vi "Replace Nested Parenthesis Pairs.vi"(6 "Existing Variables":string[](array[string]), 8 "Error In":errorcluster, 9 "Array of Parenthesis Pairs":cluster{"Start Index":i32, "Stop Index":i32}[](array[cluster]), 10 "New Variables":string[](array[string]), 11 "Formula String":string) -> (0 "Error Out":errorcluster, 1 "Array of Binary Formulas":T1[](array[typedef]), 2 "Replaced Strings":string[](array[string]), 3 "Formula String (simplified)":string)   [LabVIEW 2021, in "Formula.lvlib"]
uses:
  Binary Formula.ctl
  Binary Formula Step.ctl
  Binary Operator.ctl
  Formula.lvlib
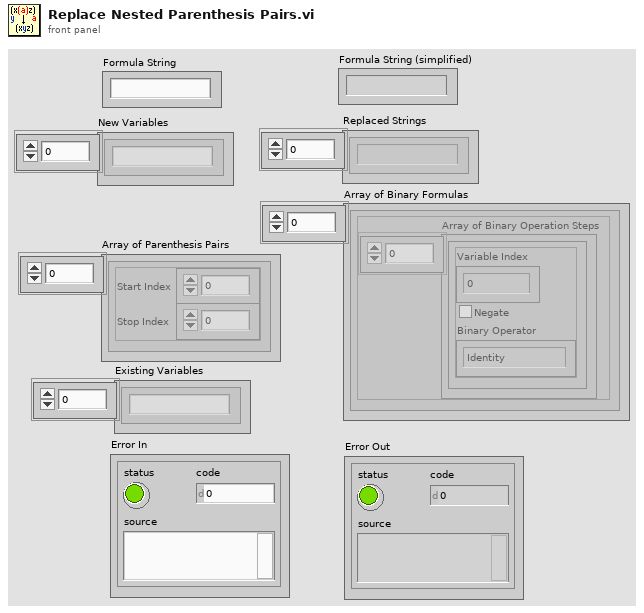
[diagram p1: front panel]
types:
  T1 = typedef "Formula.lvlib/Binary Formula.ctl" = cluster{"Array of Binary Operation Steps":T2[]}
  T2 = typedef "Formula.lvlib/Binary Formula Step.ctl" = cluster{"Variable Index":i32, "Negate":bool, "Binary Operator":T3}
  T3 = typedef "Formula.lvlib/Binary Operator.ctl" = enum16{"Identity", "AND", "OR"}
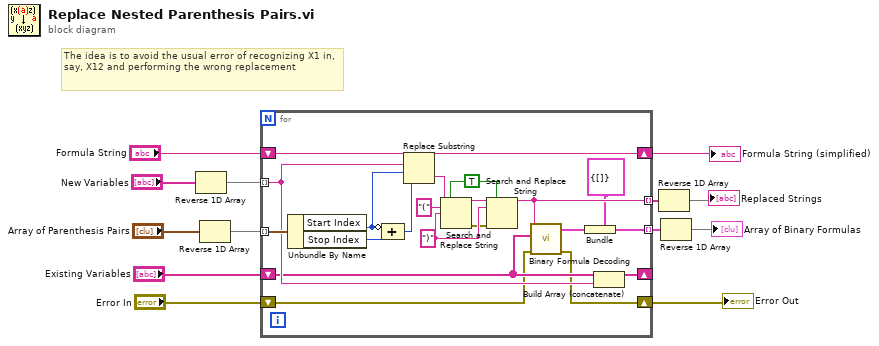
[diagram p0: block diagram]
diagram:
  # "The idea is to avoid the usual error of recognizing X1 in, say, X12 and performing the wrong replacement"
  n1 = Reverse 1D Array(array="New Variables") -> (reversed array=w8:string[])
  n2 = Reverse 1D Array(array="Array of Parenthesis Pairs") -> (reversed array=w12:cluster{"Start Index":i32, "Stop Index":i32}[])
  n3 = for {
    tunnel: w12 -> [w34] mode=indexing
    shift-right: [w32] -> w6
    shift-left: "Formula String" -> [w33]
    tunnel: [w20] -> w10 mode=indexing
    tunnel: w8 -> [w22] mode=indexing
    shift-right: [w21] -> _
    shift-left: "Existing Variables" -> [w19]
    shift-right: [w17] -> w3
    shift-left: "Error In" -> [w18]
    tunnel: [w14] -> w2 mode=indexing
    w23 = TRUE ("replace all? (F)")
    w25 = ")" ("replace string (\"\")")
    n4 = Unbundle By Name(w34) -> ("Start Index"=w31:i32, "Stop Index"=w30:i32)
    n5 = Compound Arithmetic op=ADD(invert w31, w30) -> (w29:i32)
    n6 = Replace Substring(2:w29, 3:w31, 4:w22, 5:w33) -> (0:w28:string, 1:w32:string)
    n7 = Search and Replace String(replace all?=w23, input string=w28, search string="(", replace string=w25) -> (result string=w26:string, error out=w24:errorcluster)  [unwired: 4 in, 2 out]
    n8 = Search and Replace String(replace all?=w23, input string=w26, search string=w25, error in=w24) -> (result string=w20:string)  [unwired: 4 in, 3 out]
    n9 = call "Binary Formula Decoding.vi"("Error In"=w18, "Variables"=w19, "Formula"=w20) -> ("Error Out"=w17:errorcluster, "Array of Binary Operation Steps"=w16:T2[])  [unwired: 7 in]
    n10 = Bundle(cluster=T1 {"Array of Binary Operation Steps"=[]} ("output cluster"), "Array of Binary Operation Steps"=w16) -> (w14:T1)
    n11 = Build Array (concatenate)(w19, w22) -> (w21:string[])
  }
  "Formula String (simplified)" <- w6
  "Error Out" <- w3
  n12 = Reverse 1D Array(array=w10) -> (reversed array=→"Replaced Strings":string[])
  n13 = Reverse 1D Array(array=w2) -> (reversed array=→"Array of Binary Formulas":T1[])
